vi "state selection.vi"() -> ()   [LabVIEW 2014]
uses:
  Collector State.ctl
panel:
  in  "buttons":bool[](array[boolean])
  out "error out":errorcluster
  out "data":T1
  out "state":i32
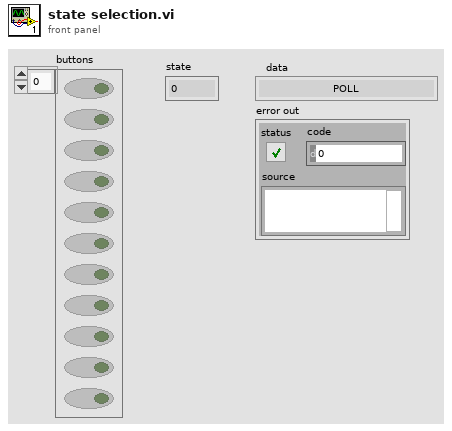
[diagram p1: front panel]
types:
  T1 = typedef "Collector State.ctl" = enum16{"POLL", "INITIALIZE", "V50 Report or GET Record", "VsVr Report", "SAVE SHOTS", "ADD SHOT", "CLEAR SHOTS", "NEXT SHOT", "DELETE SHOT", "READY CLOCK", "PROC SHOTS", "CHECK DAQ"}
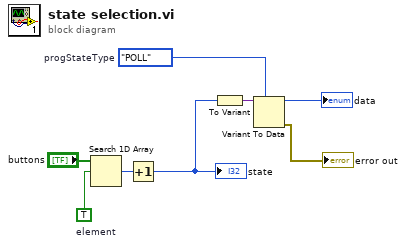
[diagram p0: block diagram]
diagram:
  w4 = TRUE  # element
  w8 = Collector_State."POLL"  # progStateType
  n1 = Search 1D Array(1D array="buttons", element=w4) -> (index of element=w3:i32)  [unwired: 1 out]
  n2 = Increment(x=w3) -> (x+1=w1:i32)
  "state" <- w1
  n3 = To Variant(anything=w1) -> (Variant=w7:variant)
  n4 = Variant To Data(type=w8, Variant=w7) -> (data=→"data":T1, error out=→"error out":errorcluster)  [unwired: 1 in]
